vi "PH_VacuumControl.evt Set Fit Starts MT.vi"(0 "i ref in":refnum<vi>, 1 "Instance":string="N/A", 2 "Start Fit MT":dbl(ring) items=["1"=0.0, "2"=1.0, "3"=2.0, "6"=5.0, "7"=6.0], 3 "Continue Fit MT":dbl=2.0, 5 "error in (no error)":errorcluster) -> (14 "i ref out":refnum<vi>, 19 "error out":errorcluster)   [LabVIEW 2014, in "PH_VacuumControl.lvlib"]
doc: "This VI calls the Proc Case to set the Fit Start value."
uses:
  PH_VacuumControl.lvlib
  CS_Core/CSSystem/CoreLib/CoreLib.double 2 byte array.vi
  CS_Core/CSSystem/CoreLib/CoreLib.lvlib
  CS_Core/BaseProcess/BaseProcess.lvlib
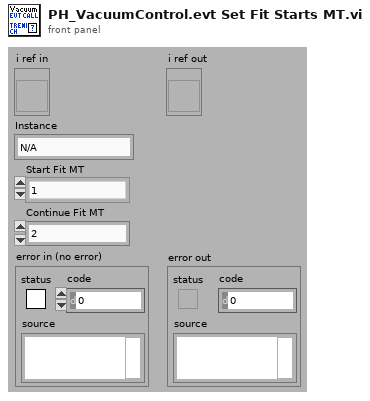
[diagram p1: front panel]
types:
  T1 = typedef "CoreDefs.rawDataType.ctl" = i8[]
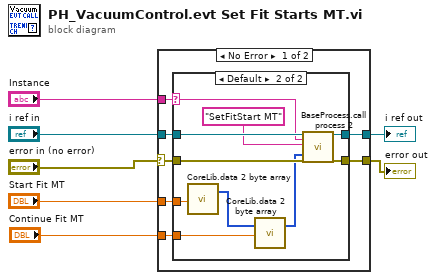
[diagram p0: block diagram]
diagram:
  n1 = case shown="No Error" "error in (no error)" {
    selector: "error in (no error)" -> [w9 w27]
    tunnel: [w14 w28] -> w7
    tunnel: [w13 w27] -> w6
    tunnel: "i ref in" -> [w12 w28]
    tunnel: "Instance" -> [w11 _]
    tunnel: "Start Fit MT" -> [w10 _]
    tunnel: "Continue Fit MT" -> [w8 _]
    frame No Error {
      n2 = case shown="Default" w11 {
        selector: w11 -> [_ w22]
        tunnel: [w16 w26] -> w14
        tunnel: [w15 w25] -> w13
        tunnel: w12 -> [w16 w24]
        tunnel: w9 -> [w15 w23]
        tunnel: w10 -> [_ w20]
        tunnel: w8 -> [_ w17]
        frame "N/A" {
        }
        frame Default {
          n3 = call-poly "CoreLib.data 2 byte array.vi"("f64"=w20) -> ("byteArray out"=w19:T1)  [unwired: 18 in]
          n4 = call-poly "CoreLib.data 2 byte array.vi"("byteArray"=w19, "f64"=w17) -> ("byteArray out"=w18:T1)  [unwired: 17 in]
          n5 = call "BaseProcess.call process 2.vi"("i ref in"=w24, "Object"=w22, "Selector"="SetFitStart MT", "Data"=w18, "error in (no error)"=w23) -> ("i ref out"=w26:refnum<vi>, "error out"=w25:errorcluster)  [unwired: 13 in]
        }
      }
    }
    frame Error {
    }
  }
  "error out" <- w6
  "i ref out" <- w7
